vi "BuildMenuRuntime.vi"(0 "XRef":T19, 1 "Point":T17, 2 "State In":T8) -> (14 "Menu Specification":T2, 15 "Fatal Error Out":T1)   [LabVIEW 2020, in "FlexBlock.xnode"]
uses:
  FlexBlock.xnode
  <vilib>/XNodeSupport/XNodeXNodeRef.ctl
  <vilib>/XNodeSupport/XNodePoint.ctl
  <vilib>/XNodeSupport/XNodeInt.ctl
  State.ctl
  <vilib>/XNodeSupport/XNodeMenuSpecs3.ctl
  <vilib>/XNodeSupport/XNodeMenuSpec3.ctl
  <vilib>/XNodeSupport/XNodeString.ctl
  <vilib>/XNodeSupport/XNodeBool.ctl
  <vilib>/XNodeSupport/XNodeStandardHelpInfo.ctl
  <vilib>/XNodeSupport/XNodePath.ctl
  <vilib>/XNodeSupport/XNodeErrorCluster.ctl
  <vilib>/XNodeSupport/NI_XNodeSupport.lvlib
  FlexBlocks/Terminal Direction.ctl
  FlexBlocks/FlexBlocks.lvlib
  FlexBlocks/Value Mode.ctl
  FlexBlocks/Terminal State.ctl
  FlexBlocks/Type Descriptor.ctl
  FlexBlocks/Errors.ctl
  <vilib>/picture/picture.llb/imagedata.ctl
  FlexBlocks/Special Terminal.ctl
  FlexBlocks/Calculated Sizes.ctl
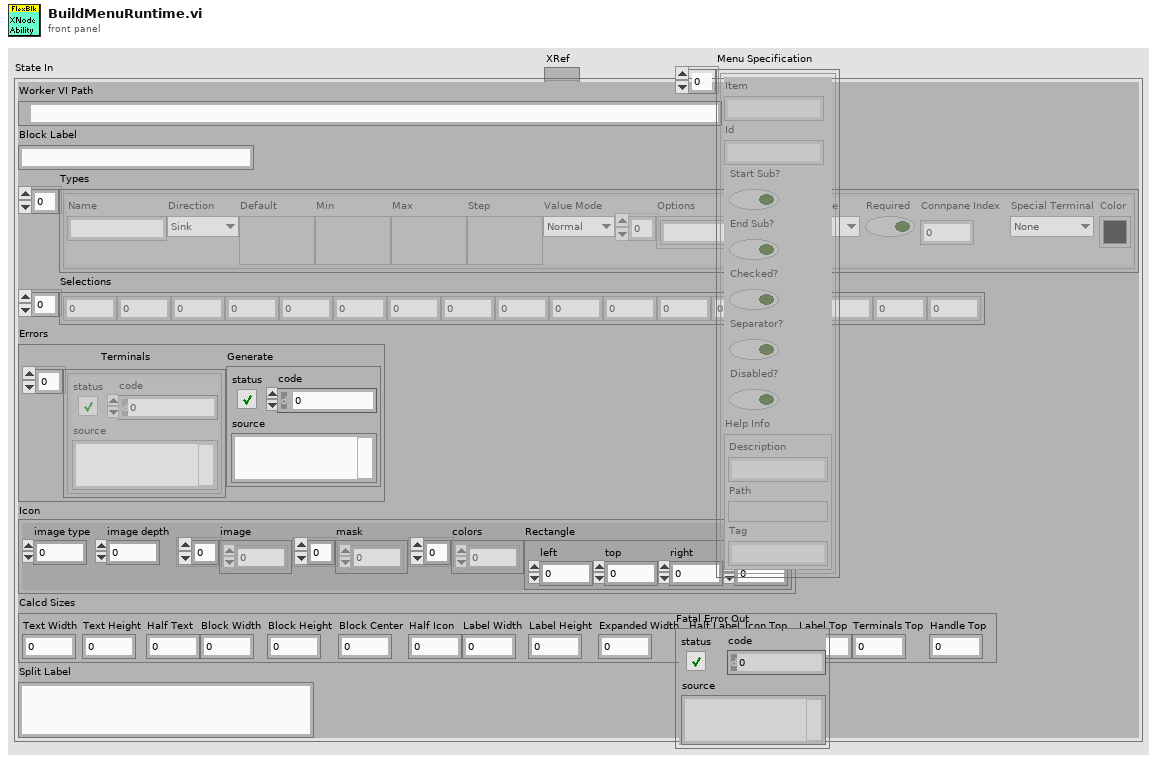
[diagram p1: front panel]
types:
  T1 = typedef "NI_XNodeSupport.lvlib/XNodeErrorCluster.ctl" = errorcluster
  T2 = typedef "NI_XNodeSupport.lvlib/XNodeMenuSpecs3.ctl" = T3[]
  T3 = typedef "NI_XNodeSupport.lvlib/XNodeMenuSpec3.ctl" = cluster{"Item":T4, "Id":T4, "Start Sub?":T5, "End Sub?":T5, "Checked?":T5, "Separator?":T5, "Disabled?":T5, "Help Info":T6}
  T4 = typedef "NI_XNodeSupport.lvlib/XNodeString.ctl" = string
  T5 = typedef "NI_XNodeSupport.lvlib/XNodeBool.ctl" = bool
  T6 = typedef "NI_XNodeSupport.lvlib/XNodeStandardHelpInfo.ctl" = cluster{"Description":T4, "Path":T7, "Tag":T4}
  T7 = typedef "NI_XNodeSupport.lvlib/XNodePath.ctl" = path
  T8 = typedef "FlexBlock.xnode/State.ctl" = cluster{"Worker VI Path":path, "Block Label":string, "Types":T9[], "Selections":i32[], "Errors":T14, "Icon":T15, "Calcd Sizes":T16, "Split Label":string}
  T9 = typedef "FlexBlocks.lvlib/Type Descriptor.ctl" = cluster{"Name":string, "Direction":T10, "Default":variant, "Min":variant, "Max":variant, "Step":variant, "Value Mode":T11, "Options":string[], "Terminal State":T12, "Required":bool, "Connpane Index":i32, "Special Terminal":T13, "Color":u32}
  T10 = typedef "FlexBlocks.lvlib/Terminal Direction.ctl" = enum16{"Sink", "Source"}
  T11 = typedef "FlexBlocks.lvlib/Value Mode.ctl" = enum16{"Normal", "Range", "Select"}
  T12 = typedef "FlexBlocks.lvlib/Terminal State.ctl" = enum16{"Unwired", "BadType", "BadRef", "Channel", "Value", "Control Ref"}
  T13 = typedef "FlexBlocks.lvlib/Special Terminal.ctl" = enum16{"None", "Action", "Init", "Tag", "State in", "State out", "Error"}
  T14 = typedef "FlexBlocks.lvlib/Errors.ctl" = cluster{"Terminals":errorcluster[], "Generate":errorcluster}
  T15 = typedef "imagedata.ctl" = cluster{"image type":i32, "image depth":i32, "image":u8[], "mask":u8[], "colors":u32[], "Rectangle":cluster{"left":i16, "top":i16, "right":i16, "bottom":i16}}
  T16 = typedef "FlexBlocks.lvlib/Calculated Sizes.ctl" = cluster{"Text Width":i32, "Text Height":i32, "Half Text":i32, "Block Width":i32, "Block Height":i32, "Block Center":i32, "Half Icon":i32, "Label Width":i32, "Label Height":i32, "Expanded Width":i32, "Half Label":i32, "Icon Top":i32, "Label Top":i32, "Terminals Top":i32, "Handle Top":i32}
  T17 = typedef "NI_XNodeSupport.lvlib/XNodePoint.ctl" = cluster{"H":T18, "V":T18}
  T18 = typedef "NI_XNodeSupport.lvlib/XNodeInt.ctl" = i32
  T19 = typedef "NI_XNodeSupport.lvlib/XNodeXNodeRef.ctl" = refnum<vi>
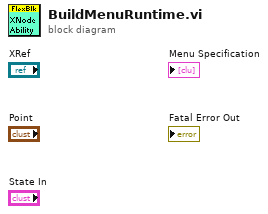
[diagram p0: block diagram]
diagram:
